vi "Frame Counter.vi"(8 "Error In":errorcluster) -> (0 "Error Out":errorcluster, 3 "Frame Count":u64)   [LabVIEW 2021, in "Display Manager.lvclass"]
uses:
  Display Manager.lvclass
  Display Manager.lvclass/Display Manager.ctl
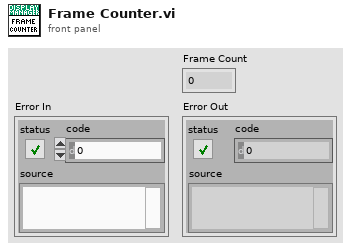
[diagram p1: front panel]
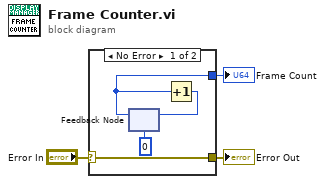
[diagram p0: block diagram]
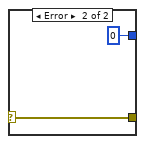
[diagram p2: hidden frame]
diagram:
  n1 = case shown="No Error" "Error In" {
    selector: "Error In" -> [w4 w8]
    tunnel: [w6 u64 0] -> w3
    tunnel: [w4 w8] -> w1
    frame No Error {
      n2 = feedback #1(u64 0) -> (w6:u64)
      n3 = Increment(x=w6) -> (x+1=w7:u64)
      n4 = feedback-in #1(w7) -> ()
    }
    frame Error {
    }
  }
  "Frame Count" <- w3
  "Error Out" <- w1
